vi "Start Log.vi"(8 "error in (no error)":errorcluster, 9 "Timestamp":string, 10 "Series":string, 11 "LoggingAPI in":refnum<class "LoggingAPI.lvclass">) -> (0 "error out":errorcluster, 3 "LoggingAPI out":refnum<class "LoggingAPI.lvclass">)   [LabVIEW 2020, in "Volatus.lvlib" / "LoggingAPI.lvclass"]
uses:
  LoggingAPI.lvclass
  LoggingAPI.lvclass/LoggingAPI.ctl
  LoggingManager Messages/Start Log Msg/Start Log Msg.lvclass/Start Log Msg.ctl
  <vilib>/ActorFramework/Message Enqueuer/Message Enqueuer.lvclass/Message Enqueuer.ctl
  <vilib>/ActorFramework/Message Enqueuer/Enqueue.vi
  LoggingManager Messages/Start Log Msg/Start Log Msg.lvclass
  C:/Program Files (x86)/National Instruments/LabVIEW 2020/vi.lib/ActorFramework/Message/Message.lvclass
  <vilib>/ActorFramework/Message Priority Queue/Priority Enqueue.vi
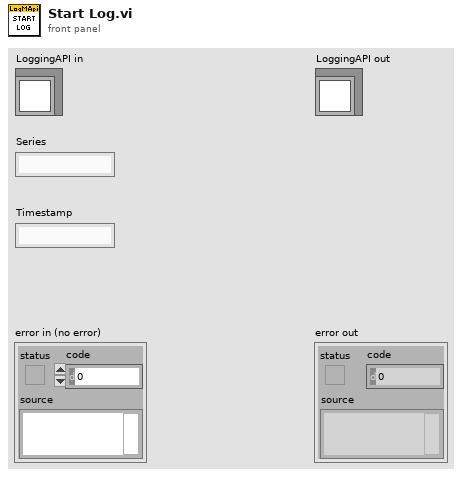
[diagram p1: front panel]
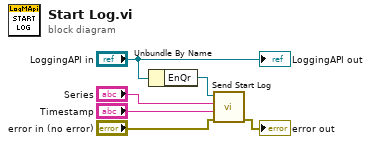
[diagram p0: block diagram]
diagram:
  n1 = Unbundle By Name("LoggingAPI in") -> ("EnQr"=w5:refnum<class "Message Enqueuer.lvclass">)
  n2 = call "Send Start Log.vi"("error in (no error)"="error in (no error)", "Timestamp"="Timestamp", "Series"="Series", "Message Enqueuer"=w5) -> ("error out"=→"error out":errorcluster)  [unwired: 6 in, 1 out]
  "LoggingAPI out" <- "LoggingAPI in"
